vi "Calc_Head_Tail_Angle.vi"(7 "Body Center":cluster{"X":dbl, "Y":dbl}, 8 "Tail Angle":dbl, 9 "Tail Center":cluster{"X":dbl, "Y":dbl}, 10 "Head Angle":dbl, 11 "Head Center":cluster{"X":dbl, "Y":dbl}) -> (3 "Head-Tail Angle":dbl)   [LabVIEW 2014]
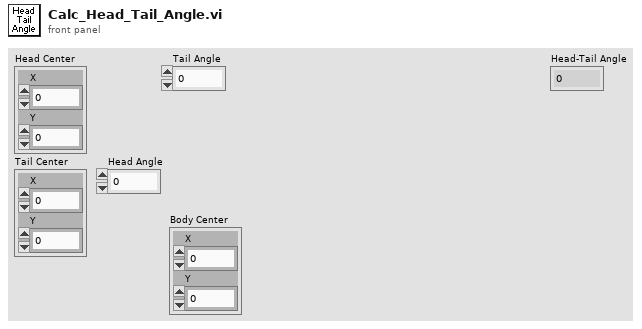
[diagram p1: front panel]
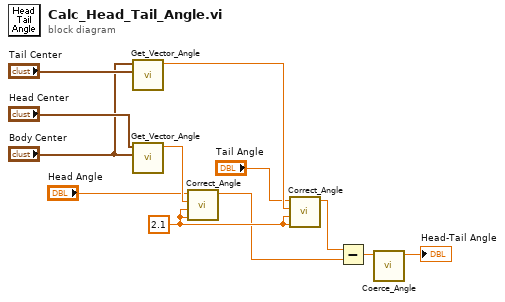
[diagram p0: block diagram]
diagram:
  w10 = 2.1 ("Inverse Th")
  n1 = call "Get_Vector_Angle.vi"("End Point"="Tail Center", "Start Point"="Body Center") -> ("Angle Out"=w12:dbl)  [unwired: 9 in]
  n2 = call "Get_Vector_Angle.vi"("End Point"="Body Center", "Start Point"="Head Center") -> ("Angle Out"=w11:dbl)  [unwired: 9 in]
  n3 = call "Correct_Angle.vi"("Keep Tgt Th"=w10, "Inverse Th"=w10, "Tgt Angle"=w11, "Src Angle"="Head Angle") -> ("Output Angle"=w1:dbl)  [unwired: 7 in]
  n4 = call "Correct_Angle.vi"("Keep Tgt Th"=w10, "Inverse Th"=w10, "Tgt Angle"=w12, "Src Angle"="Tail Angle") -> ("Output Angle"=w2:dbl)  [unwired: 7 in]
  n5 = Subtract(x=w2, y=w1) -> (x-y=w9:dbl)
  n6 = call "Coerce_Angle.vi"("In Angle"=w9) -> ("Out Angle"=→"Head-Tail Angle":dbl)  [unwired: 10 in]
